vi "TangoGroupCommandInOutTest.vi"() -> ()   [LabVIEW 2014, in "examples.lvlib"]
uses:
  vis/tango_vi.llb/fromDevDouble.vi
  vis/tango_vi.llb/toDevULong64.vi
  examples.lvlib
  vis/tango_vi.llb/tango.lvlib
panel:
  out "output value from dev-3 in the group":dbl
  out "output value from dev-2 in the group":dbl
  out "output value from dev-1 in the group":dbl
  out "T.Grp.W Error":errorcluster caption="T.Grp.Cmd Error"
  in  "command to exec. on the group":string="DevDouble"
  in  "input value for dev-1 in the group":dbl=1.1
  in  "input value for dev-2 in the group":dbl=2.2
  in  "input value for dev-3 in the group":dbl=3.3
  in  "ignored devices":string[](array[string])
  in  "managed devices":string[](array[string])=["tango/tangotest/1", "tango/tangotest/2", "tango/tangotest/3"]
  in  "group name":string="w_test_group"
  out "group id":i32
  # "TANGO  Binding for LabVIEW - WriteAttributes example"
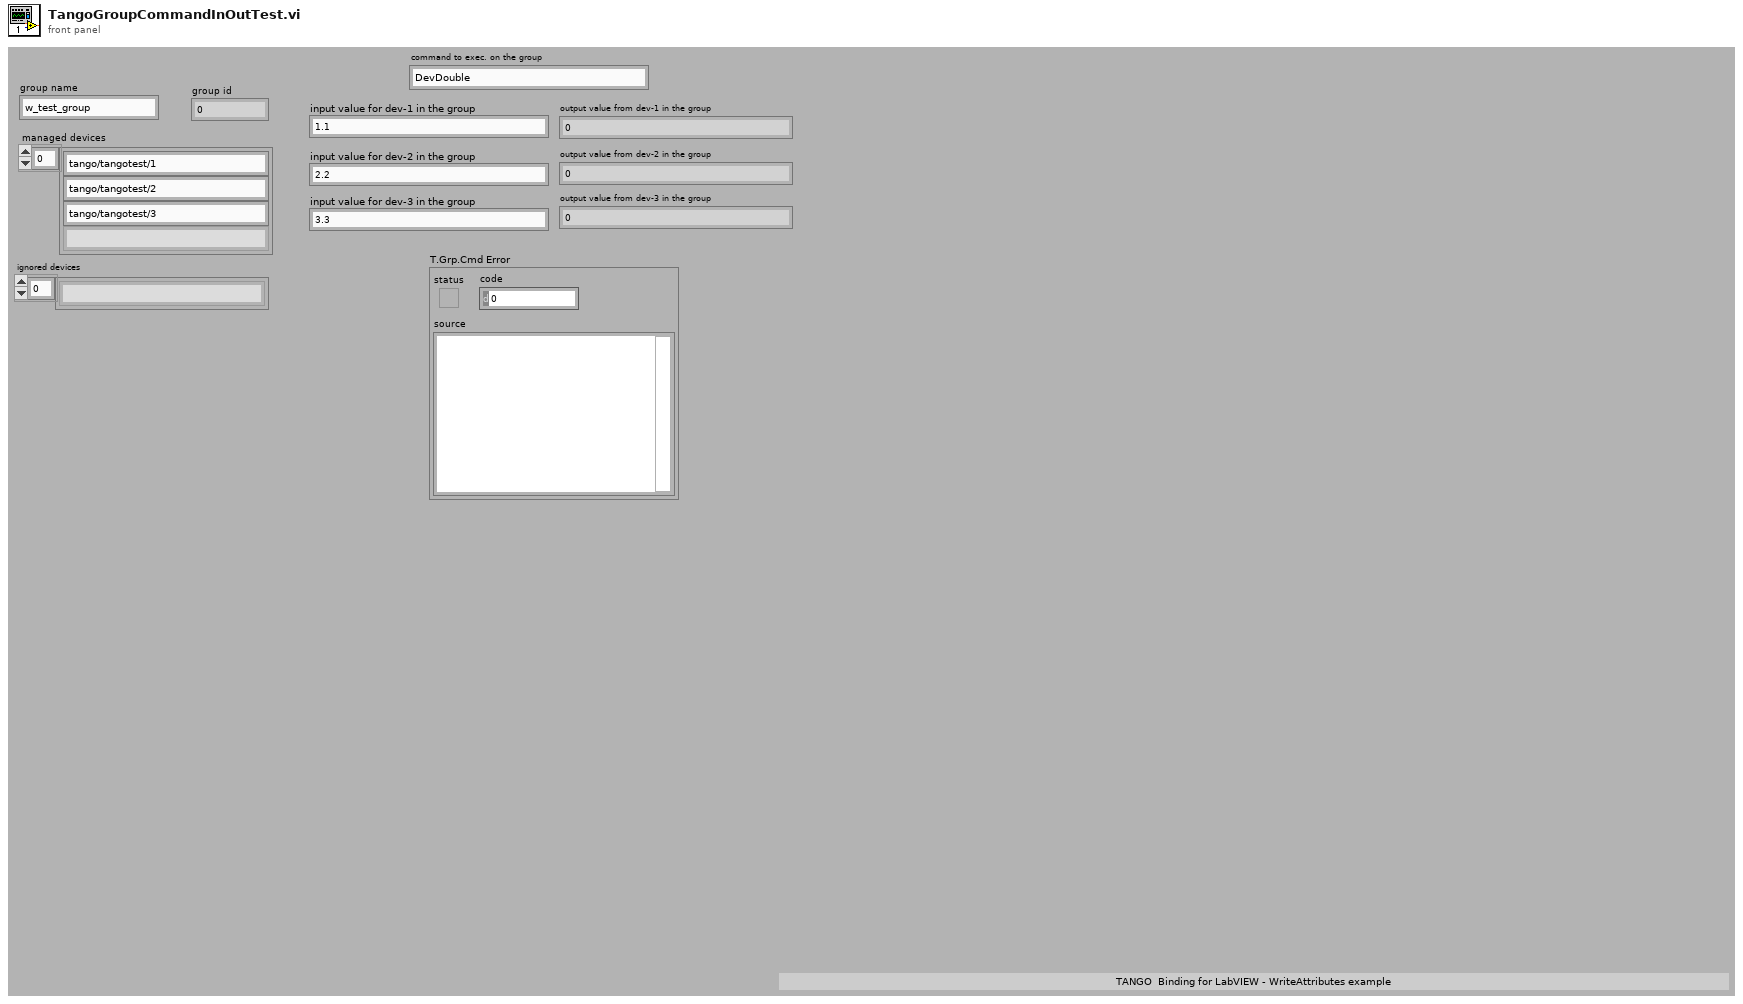
[diagram p1: front panel]
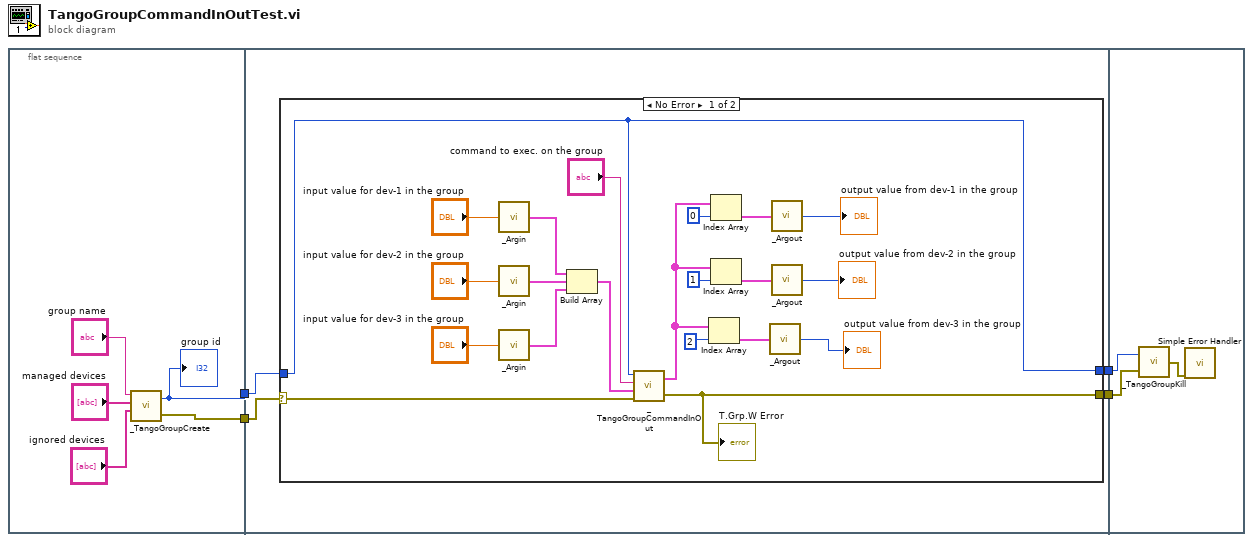
[diagram p0: block diagram]
diagram:
  n1 = flat-sequence {
    tunnel: [w8] -> w4
    tunnel: [w7] -> w3
    tunnel: w4 -> [w11]
    tunnel: [w10] -> w2
    tunnel: w3 -> [w13]
    tunnel: [w12] -> w1
    tunnel: w2 -> [w39]
    tunnel: w1 -> [w38]
    frame #0 {
      n2 = call "_TangoGroupCreate.vi"("ignored devices"="ignored devices", "managed devices"="managed devices", "group name"="group name") -> ("error out"=w7:errorcluster, "group id"=w8:i32)  [unwired: 1 in]
      "group id" <- w8
    }
    frame #1 {
      n3 = case shown="No Error" w13 {
        selector: w13 -> [w27 w36]
        tunnel: w11 -> [w31 w35]
        tunnel: [w18 w36] -> w12
        tunnel: [w31 w35] -> w10
        frame No Error {
          n4 = call-poly "_Argin.vi"("argin"="input value for dev-1 in the group") -> ("ArgIO"=w29:cluster{"num data":u8[], "str data":string[]})
          n5 = call-poly "_Argin.vi"("argin"="input value for dev-2 in the group") -> ("ArgIO"=w30:cluster{"num data":u8[], "str data":string[]})
          n6 = call-poly "_Argin.vi"("argin"="input value for dev-3 in the group") -> ("ArgIO"=w28:cluster{"num data":u8[], "str data":string[]})
          n7 = Build Array(w29, w30, w28) -> (w26:cluster{"num data":u8[], "str data":string[]}[])
          n8 = call "_TangoGroupCommandInOut.vi"("error in"=w27, "args_in"=w26, "command_name"="command to exec. on the group", "group id"=w31) -> ("error out"=w18:errorcluster, "args_out"=w17:cluster{"num data":u8[], "str data":string[]}[])
          "T.Grp.W Error" <- w18
          n9 = Index Array(array=w17, index=2 ("indice")) -> (element=w21:cluster{"num data":u8[], "str data":string[]})
          n10 = Index Array(array=w17, index=0 ("indice")) -> (element=w22:cluster{"num data":u8[], "str data":string[]})
          n11 = Index Array(array=w17, index=1 ("indice")) -> (element=w20:cluster{"num data":u8[], "str data":string[]})
          n12 = call-poly "_Argout.vi"("ArgIO"=w21) -> ("argout"=→"output value from dev-3 in the group":u64)
          n13 = call-poly "_Argout.vi"("ArgIO"=w22) -> ("argout"=→"output value from dev-1 in the group":u64)
          n14 = call-poly "_Argout.vi"("ArgIO"=w20) -> ("argout"=→"output value from dev-2 in the group":u64)
        }
        frame Error {
        }
      }
    }
    frame #2 {
      n15 = call "_TangoGroupKill.vi"("error in"=w38, "group id"=w39) -> ("error out"=w37:errorcluster)
      n16 = call <vilib>:"Simple Error Handler.vi"("error in (no error)"=w37) -> ()  [unwired: 4 in, 5 out]
    }
  }
